vi "Get Target Address.vi"(8 "error in (no error)":errorcluster, 11 "calling VI location":path) -> (0 "error out":errorcluster, 3 "target address":string)   [LabVIEW 2020]
uses:
  niveristand-custom-device-testing-tools/VeriStandTestUtilities/VeriStandTestUtilities.lvlib
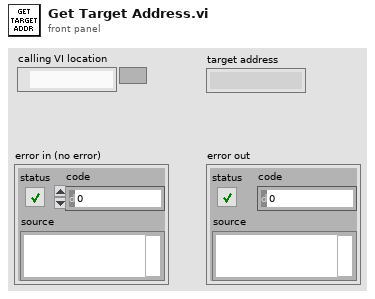
[diagram p1: front panel]
types:
  T1 = typedef "VeriStandTestUtilities.lvlib/TargetsConfiguration.ctl" = cluster{"Supported Targets":cluster{"IP Address / Hostname":string, "Target Platform":T2}[], "Active Configuration":T2}
  T2 = typedef "VeriStandTestUtilities.lvlib/TargetPlatform.ctl" = enum16{"Windows", "Linux64CRIO", "Linux64PXI", "LinuxARM", "PharLap"}
  T3 = cluster{"IP Address / Hostname":string, "Target Platform":T2}[]
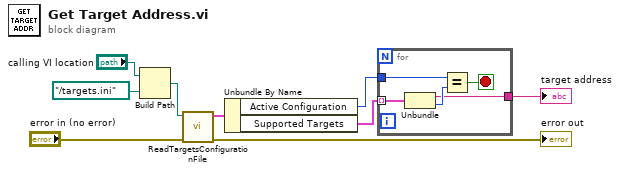
[diagram p0: block diagram]
diagram:
  n1 = Build Path(base path="calling VI location", name or relative path=path "../targets.ini" ("Hardware File Path")) -> (appended path=w8:path)
  n2 = call "ReadTargetsConfigurationFile.vi"("error in (no error)"="error in (no error)", "targets.ini file"=w8) -> ("error out"=→"error out":errorcluster, "Targets Configuration"=w9:T1)  [unwired: 8 in]
  n3 = Unbundle By Name(w9) -> ("Active Configuration"=w3:T2, "Supported Targets"=w4:T3)
  n4 = for {
    tunnel: w4 -> [w14] mode=indexing
    tunnel: w3 -> [w13]
    tunnel: [w10] -> w2
    stop <- w12 stop-if-true
    n5 = Unbundle(w14) -> ("IP Address / Hostname"=w10:string, "Target Platform"=w11:T2)
    n6 = Equal?(x=w13, y=w11) -> (x = y?=w12:bool)
  }
  "target address" <- w2
